vi "Motor to Joystick.vi"(8 "Drive Motor":dbl, 11 "Rotational Motor":dbl) -> (0 "Joy Y":dbl, 3 "Joy X":dbl)   [LabVIEW 2014]
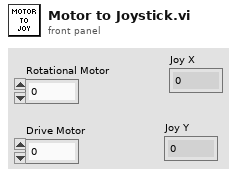
[diagram p1: front panel]
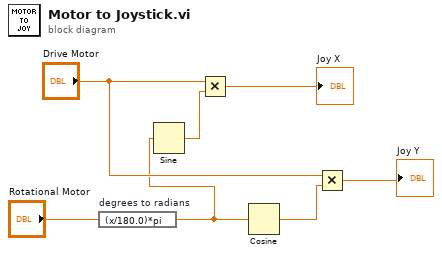
[diagram p0: block diagram]
diagram:
  n1 = expression code="(x/180.0)*pi" "degrees to radians"("Rotational Motor") -> (w4:dbl)
  n2 = Sine(x=w4) -> (sin(x)=w3:dbl)
  n3 = Multiply(x="Drive Motor", y=w3) -> (x*y=→"Joy X":dbl)
  n4 = Cosine(x=w4) -> (cos(x)=w5:dbl)
  n5 = Multiply(x="Drive Motor", y=w5) -> (x*y=→"Joy Y":dbl)
